vi "MS SQL_InRFID_STN40.vi"(7 "OP20B_004_PREACTUATION":T1, 8 "error in (no error)":errorcluster, 10 "RFID":string, 11 "Ref in":T2={"MS SQL Connection"=refnum, "UDL File"=path "", "Time"="", "DCODE"="", "WIP+1"=0, "MC No?"=0, "POKAYOKE?"=FALSE, "Expected Result"="", "Result [Status]"="", "Clock"=0.0, "RFID"="", "WIP Queue"=refnum, "TS Parameter"={"ProfitCenterCode"="", "LineCode"="", "WorkOrderNumber"="", "Model"="", "Model_with_Prefix"="", "VendorCode"="", "SetParameterDateCode"="", "PokaYoke"=0, "Target"=1, "Live_DateCode"="", "CustomerPartNumber"="", "Hand"="", "Ent_Stamp"=timestamp(0 s since 1904-01-01), "STS_CD"=0.0}, "Data_Queue"=[], "RFID Serial No."=""} {"TS Parameter"."Target" min=1 max=100000; "TS Parameter"."PokaYoke" min=0 max=1}) -> (0 "error out":errorcluster, 1 "Message":picture, 3 "Ref Out out":T2={"MS SQL Connection"=refnum, "UDL File"=path "", "Time"="", "DCODE"="", "WIP+1"=0, "MC No?"=0, "POKAYOKE?"=FALSE, "Expected Result"="", "Result [Status]"="", "Clock"=0.0, "RFID"="", "WIP Queue"=refnum, "TS Parameter"={"ProfitCenterCode"="", "LineCode"="", "WorkOrderNumber"="", "Model"="", "Model_with_Prefix"="", "VendorCode"="", "SetParameterDateCode"="", "PokaYoke"=0, "Target"=1, "Live_DateCode"="", "CustomerPartNumber"="", "Hand"="", "Ent_Stamp"=timestamp(0 s since 1904-01-01), "STS_CD"=0.0}, "Data_Queue"=[], "RFID Serial No."=""} {"TS Parameter"."Target" min=1 max=100000; "TS Parameter"."PokaYoke" min=0 max=1})   [LabVIEW 2020]
uses:
  Controls/TD SQL.ctl
  <vilib>/addons/database/Connection.llb/Conn ObjectReference.ctl
  Controls/WIP_State.ctl
  Controls/TS_Parameter.ctl
  Controls/OP20B_DataCluster.ctl
  <vilib>/addons/database/NI_Database_API.lvlib
panel:
  out "resulting string":string
  # "OP40"
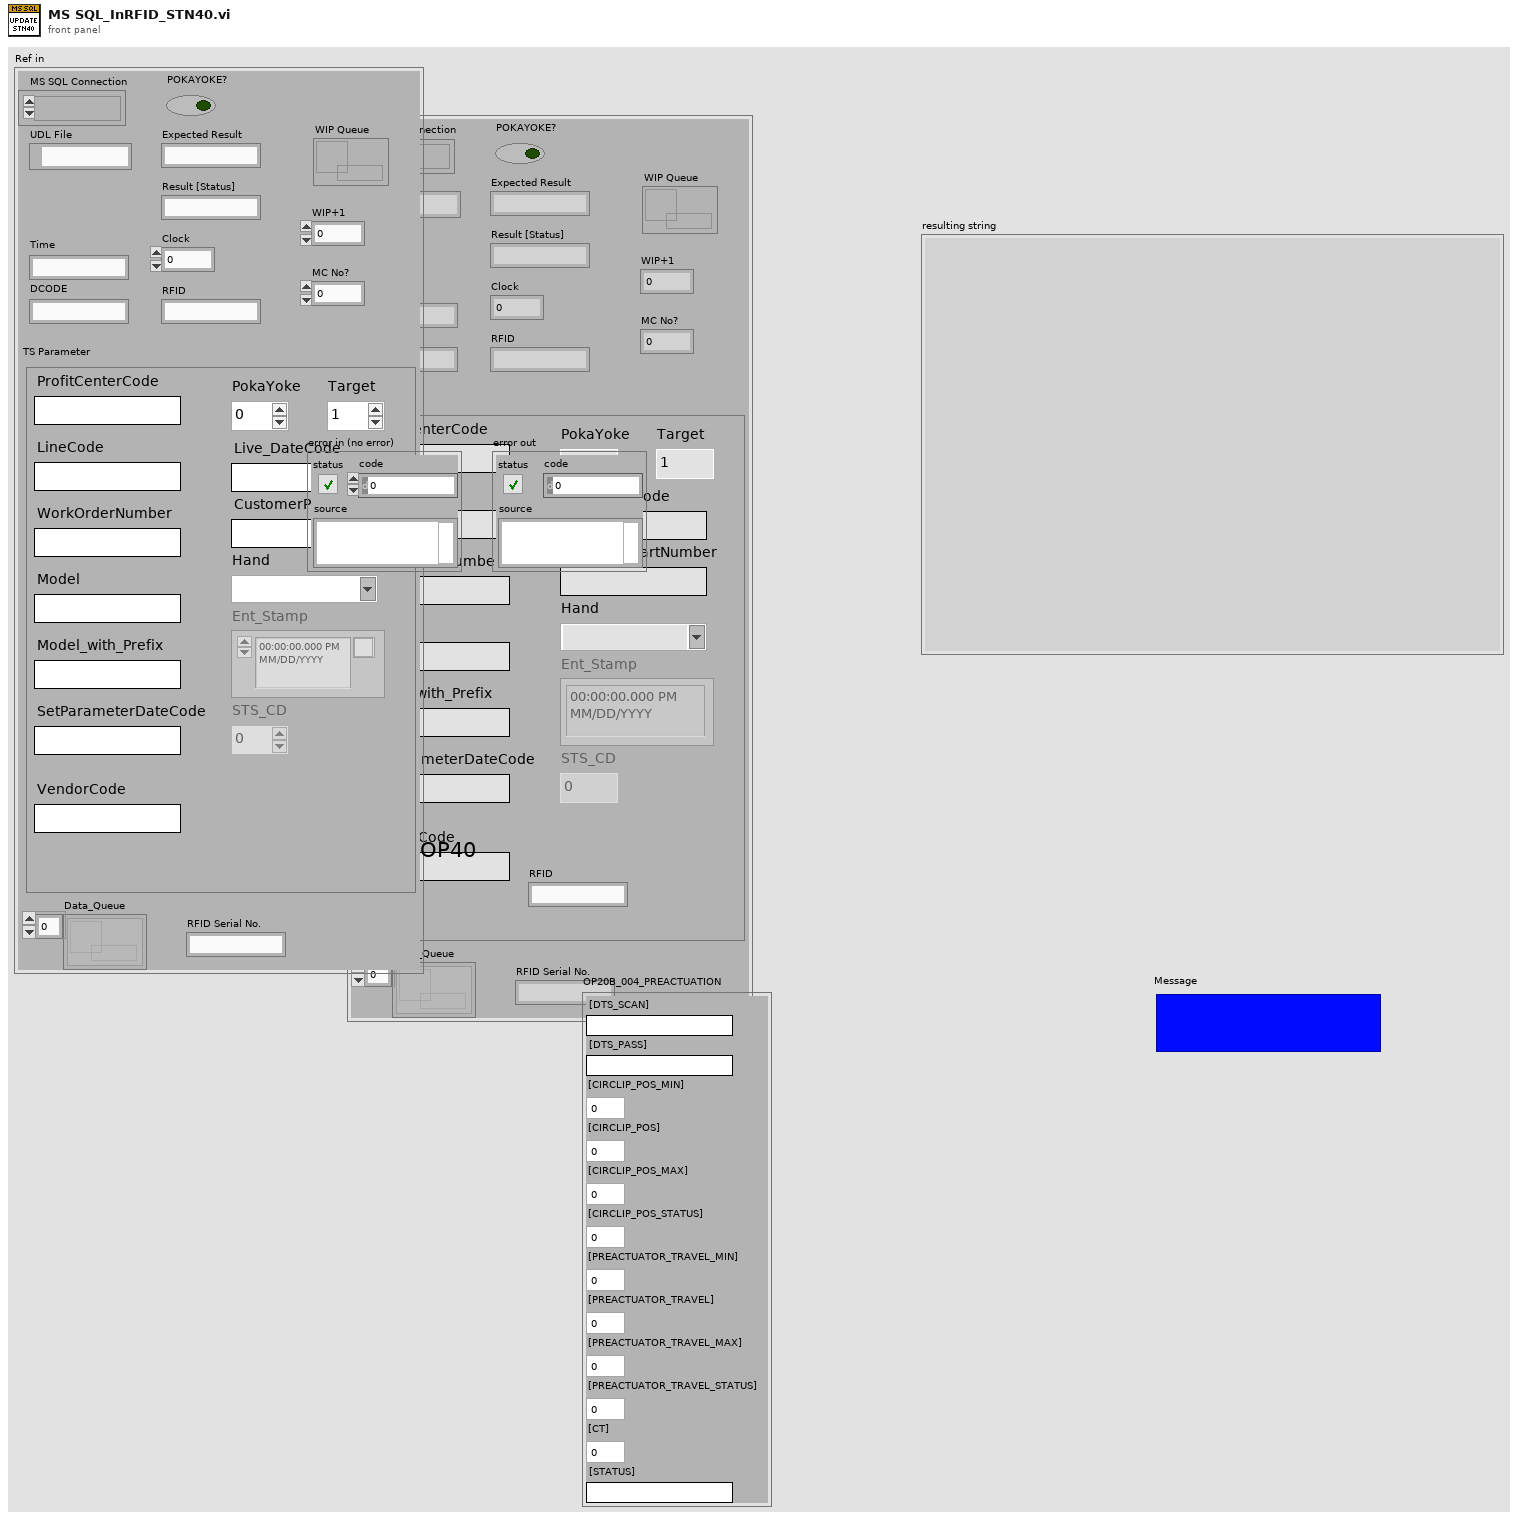
[diagram p1: front panel]
types:
  T1 = typedef "OP20B_DataCluster.ctl" = cluster{"[DTS_SCAN]":string, "[DTS_PASS]":string, "[CIRCLIP_POS_MIN]":dbl, "[CIRCLIP_POS]":dbl, "[CIRCLIP_POS_MAX]":dbl, "[CIRCLIP_POS_STATUS]":dbl, "[PREACTUATOR_TRAVEL_MIN]":dbl, "[PREACTUATOR_TRAVEL]":dbl, "[PREACTUATOR_TRAVEL_MAX]":dbl, "[PREACTUATOR_TRAVEL_STATUS]":dbl, "[CT]":dbl, "[STATUS]":string}
  T2 = typedef "TD SQL.ctl" = cluster{"MS SQL Connection":T3, "UDL File":path, "Time":string, "DCODE":string, "WIP+1":i64, "MC No?":i32, "POKAYOKE?":bool, "Expected Result":string, "Result [Status]":string, "Clock":dbl, "RFID":string, "WIP Queue":refnum<queue>, "TS Parameter":T4, "Data_Queue":refnum<queue>[], "RFID Serial No.":string}
  T3 = typedef "NI_Database_API.lvlib/Conn ObjectReference.ctl" = refnum<k1>
  T4 = typedef "TS_Parameter.ctl" = cluster{"ProfitCenterCode":string, "LineCode":string, "WorkOrderNumber":string, "Model":string, "Model_with_Prefix":string, "VendorCode":string, "SetParameterDateCode":string, "PokaYoke":i32, "Target":i32, "Live_DateCode":string, "CustomerPartNumber":string, "Hand":string, "Ent_Stamp":timestamp, "STS_CD":dbl}
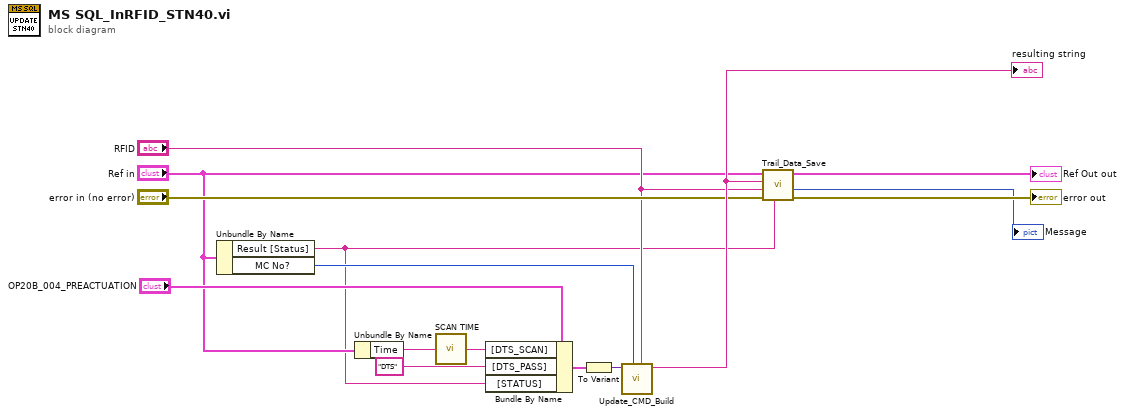
[diagram p0: block diagram]
diagram:
  n1 = Unbundle By Name("Ref in") -> ("Result [Status]"=w1:string, "MC No?"=w2:i32)
  n2 = Unbundle By Name("Ref in") -> ("Time"=w15:string)
  n3 = call "SCAN TIME.vi"("Time in"=w15) -> ("Time out"=w11:string)
  n4 = Bundle By Name(cluster="OP20B_004_PREACTUATION", "[DTS_SCAN]"=w11, "[DTS_PASS]"="DTS", "[STATUS]"=w1) -> (w14:T1)
  n5 = To Variant(anything=w14) -> (Variant=w12:variant)
  n6 = call "Update_CMD_Build.vi"("RFID"="RFID", "Machine No"=w2, "Variant"=w12) -> ("Update Query"=w9:string)  [unwired: 5 in, 1 out]
  "resulting string" <- w9
  n7 = call "Trail_Data_Save.vi"("Status"=w1, "error in (no error)"="error in (no error)", "RFID"="RFID", "Query"=w9, "Ref in"="Ref in") -> ("error out"=→"error out":errorcluster, "Message"=→"Message":picture, "Ref Out"=→"Ref Out out":T2)  [unwired: 1 in, 1 out]
